vi "SERIAL_StoreBuffer.vi"(8 "error in (no error)":errorcluster, 9 "Access Type":enum16{"set", "get", "delete"}(ring), 10 "navX Data":u8[](array[numeric]), 11 "SerialPortRef":T1) -> (0 "error out":errorcluster, 2 "navX Data":u8[](array[numeric]), 3 "SerialPortRef":T1)   [LabVIEW 2015, in "navX Library v1 (deprecated).lvlib"]
uses:
  navX Library v1 (deprecated).lvlib
  <vilib>/Rock Robotics/WPI/SerialPort/WPI_SerialPortRef.ctl
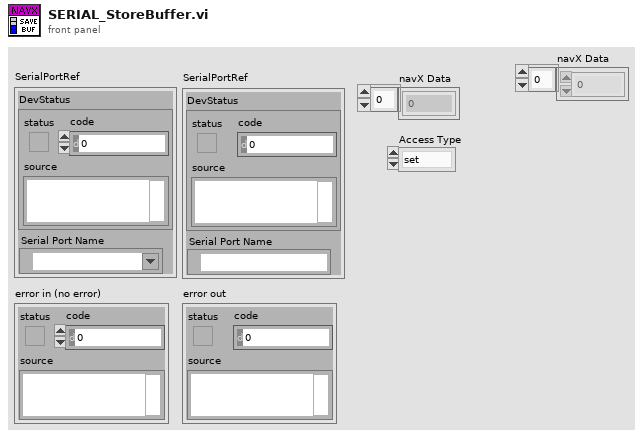
[diagram p1: front panel]
types:
  T1 = typedef "WPI_SerialPortRef.ctl" = cluster{"DevStatus":errorcluster, "Serial Port Name":refnum<visa-resource-name>}
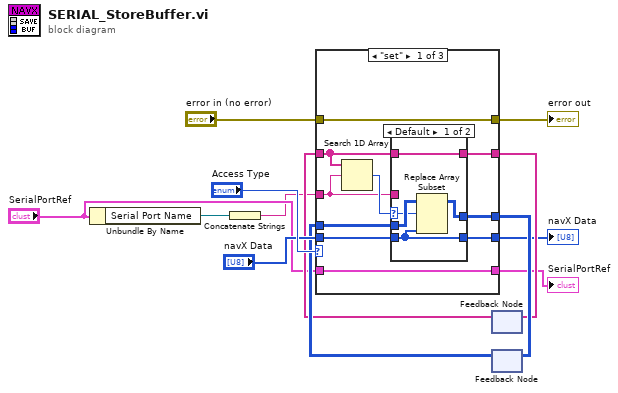
[diagram p0: block diagram]
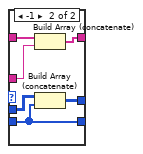
[diagram p2: hidden frame]
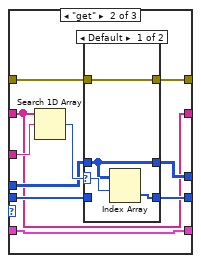
[diagram p3: hidden frame]
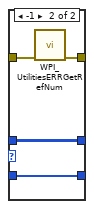
[diagram p4: hidden frame]
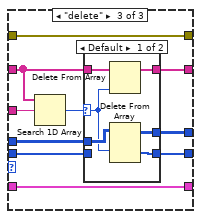
[diagram p5: hidden frame]
diagram:
  n1 = Unbundle By Name("SerialPortRef") -> ("Serial Port Name"=w9:refnum<visa-resource-name>)
  n2 = Concatenate Strings(w9) -> (w1:string)
  n3 = feedback #1() -> (w8:string[])  [unwired: 1 in]
  n4 = feedback #2() -> (w10:u8[][])  [unwired: 1 in]
  n5 = case shown="\"set\"" "Access Type" {
    tunnel: "navX Data" -> [w22 w37 w54]
    tunnel: [w21 w40 w56] -> w11
    tunnel: w10 -> [w20 w39 w55]
    tunnel: w1 -> [w16 w44 w62]
    tunnel: w8 -> [w18 w36 w59]
    tunnel: [w19 w36 w60] -> w7
    tunnel: [w14 w35 w58] -> w6
    tunnel: "SerialPortRef" -> [w14 w35 w58]
    tunnel: [w17 w41 w57] -> w4
    tunnel: "error in (no error)" -> [w17 w42 w57]
    tunnel: [w15 w38 w53] -> w2
    frame "set" {
      n6 = Search 1D Array(1D array=w18, element=w16) -> (index of element=w23:i32)  [unwired: 1 in]
      n7 = case shown="Default" w23 {
        selector: w23 -> [w24 _]
        tunnel: w22 -> [w25 w29]
        tunnel: [w28 w30] -> w21
        tunnel: w20 -> [w27 w31]
        tunnel: [w26 w32] -> w19
        tunnel: w18 -> [w26 w34]
        tunnel: w16 -> [_ w33]
        tunnel: [w25 w29] -> w15
        frame Default {
          n8 = Replace Array Subset(array=w27, new element=w25, index (row)=w24) -> (w28:u8[][])  [unwired: 1 in]
        }
        frame -1 {
          n9 = Build Array (concatenate)(w34, w33) -> (w32:string[])
          n10 = Build Array (concatenate)(w31, w29) -> (w30:u8[][])
        }
      }
    }
    frame "get" {
      n11 = Search 1D Array(1D array=w36, element=w44) -> (index of element=w43:i32)  [unwired: 1 in]
      n12 = case shown="Default" w43 {
        selector: w43 -> [w48 _]
        tunnel: w42 -> [w46 w52]
        tunnel: [w46 w51] -> w41
        tunnel: [w45 w50] -> w40
        tunnel: w39 -> [w45 w50]
        tunnel: [w47 w49] -> w38
        tunnel: w37 -> [_ w49]
        frame Default {
          n13 = Index Array(array=w45, index (row)=w48) -> (element=w47:u8[])  [unwired: 1 in]
        }
        frame -1 {
          n14 = call <vilib>:"WPI_UtilitiesERRGetRefNum.vi"("error in (no error)"=w52) -> ("ERRGetRefNum"=w51:errorcluster)  [unwired: 10 out]
        }
      }
    }
    frame "delete" {
      n15 = Search 1D Array(1D array=w59, element=w62) -> (index of element=w61:i32)  [unwired: 1 in]
      n16 = case shown="Default" w61 {
        selector: w61 -> [w66 _]
        tunnel: [w63 w71] -> w60
        tunnel: w59 -> [w68 w71]
        tunnel: [w65 w70] -> w56
        tunnel: w55 -> [w67 w70]
        tunnel: w54 -> [_ w69]
        tunnel: [w64 w69] -> w53
        frame Default {
          n17 = Delete From Array(array=w68, index=w66) -> (array with subset deleted=w63:string[])  [unwired: 1 in, 1 out]
          n18 = Delete From Array(array=w67, index (row)=w66) -> (deleted portion=w64:u8[], array with subset deleted=w65:u8[][])  [unwired: 2 in]
        }
        frame -1 {
        }
      }
    }
  }
  "navX Data" <- w2
  "error out" <- w4
  "SerialPortRef" <- w6
  n19 = feedback-in #1(w7) -> ()
  n20 = feedback-in #2(w11) -> ()
